vi "Logger Test Interface.vi"() -> ()   [LabVIEW 2012, in "Logger VIs.lvlib"]
uses:
  Logger VIs.lvlib
  State.ctl
panel:
  in  "Holding Potential":dbl(knob) scale=0.0..10.0
  in  "Current":dbl(knob) scale=0.0..10.0
  in  "Threshold":dbl(knob) scale=0.0..10.0
  in  "Resistance":dbl(knob) scale=0.0..10.0
  in  "Pressure":dbl(knob) scale=0.0..10.0
  out "Threshold":dbl(graph)
  out "Position":cluster{"X":dbl, "Y":dbl, "Z":dbl} {"Z" format="%.2f"; "Y" format="%.2f"; "X" format="%.2f"}
  out "Current State":T1=enum."LOAD"
  out "Holding Potential":dbl(graph)
  out "Pressure":dbl(graph)
  out "Current":dbl(graph)
  out "Resistance":dbl(graph)
  out "Full Path":path
  in  "base path":path
  out "error out":errorcluster
  in  "error in (no error)":errorcluster
  in  "Stop":bool caption="Start 2"
  out "Recording indicator":bool
  in  "Record":bool caption="Start 2"
  # "um"
  # "um"
  # "um"
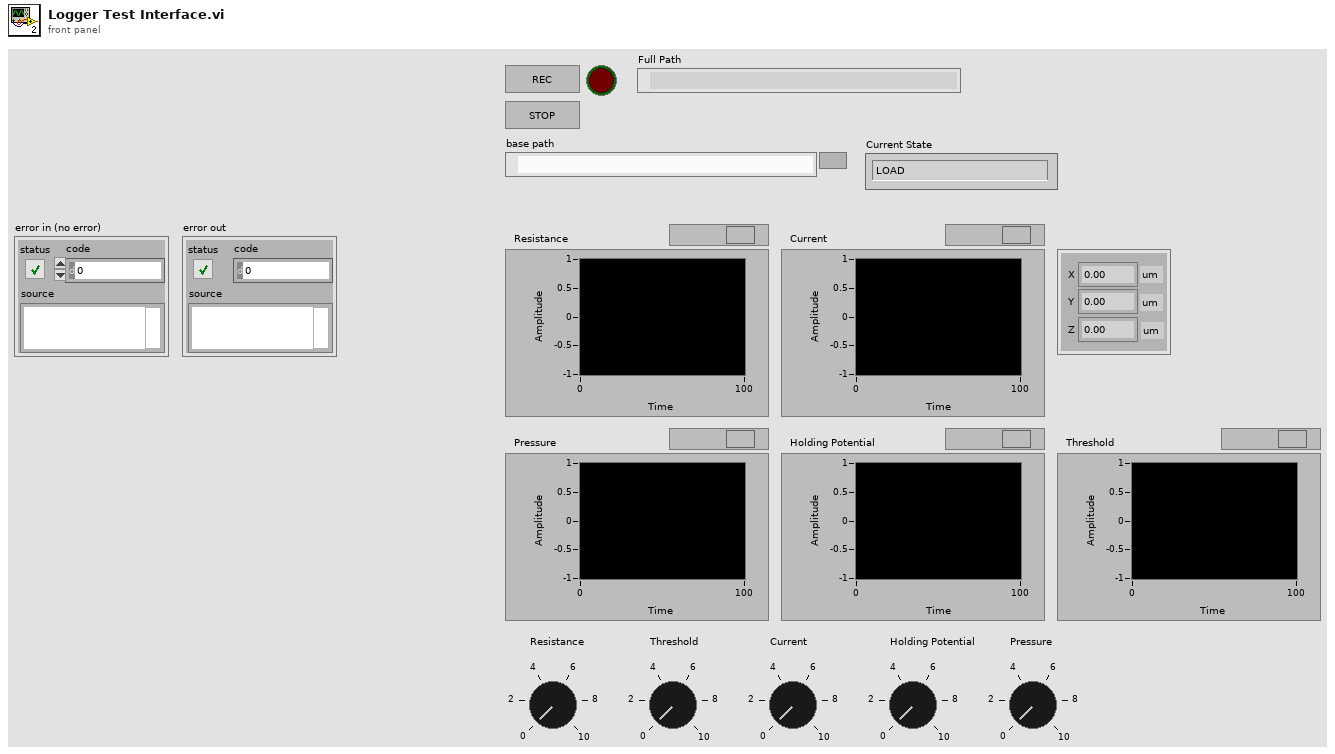
[diagram p1: front panel]
types:
  T1 = typedef "State.ctl" = enum16{"READY", "LOAD", "LOCALIZATION", "HUNTING", "SEAL", "BREAKIN", "WCR"}
  T2 = cluster{"Resistance":refnum<vi>, "Current":refnum<vi>, "Holding Potential":refnum<vi>, "Current State":refnum<vi>, "Recording indicator":refnum<vi>, "Threshold":refnum<vi>, "Pressure":refnum<vi>, "Path":refnum<vi>, "Manipulator Position":refnum<vi>}
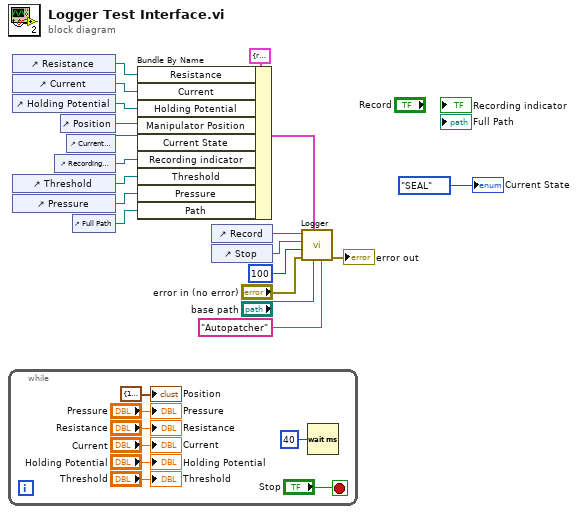
[diagram p0: block diagram]
diagram:
  n1 = while {
    stop <- "Stop" stop-if-true
    n2 = Wait (ms)(milliseconds to wait=u32 40) -> ()  [unwired: 1 out]
    "Resistance" <- "Resistance"
    "Current" <- "Current"
    "Pressure" <- "Pressure"
    "Holding Potential" <- "Holding Potential"
    "Position" <- cluster{"X":dbl, "Y":dbl, "Z":dbl} {"X"=10.0, "Y"=20.0, "Z"=30.0} ("Position")
    "Threshold" <- "Threshold"
  }
  n3 = control-ref of="Resistance"() -> (w10:refnum<vi>)
  n4 = control-ref of="Current"() -> (w9:refnum<vi>)
  n5 = control-ref of="Holding Potential"() -> (w3:refnum<vi>)
  n6 = control-ref of="Threshold"() -> (w4:refnum<vi>)
  n7 = control-ref of="Pressure"() -> (w7:refnum<vi>)
  n8 = control-ref of="Recording indicator"() -> (w8:refnum<vi>)
  n9 = control-ref of="Position"() -> (w2:refnum<vi>)
  n10 = control-ref of="Current State"() -> (w11:refnum<vi>)
  n11 = control-ref of="Full Path"() -> (w14:refnum<vi>)
  n12 = Bundle By Name(cluster=T2 {"Resistance"=refnum, "Current"=refnum, "Holding Potential"=refnum, "Current State"=refnum, "Recording indicator"=refnum, "Threshold"=refnum, "Pressure"=refnum, "Path"=refnum, "Manipulator Position"=refnum} ("Indicators"), "Resistance"=w10, "Current"=w9, "Holding Potential"=w3, "Manipulator Position"=w2, "Current State"=w11, "Recording indicator"=w8, "Threshold"=w4, "Pressure"=w7, "Path"=w14) -> (w6:T2)
  n13 = control-ref of="Record"() -> (w19:refnum<vi>)
  n14 = control-ref of="Stop"() -> (w1:refnum<vi>)
  n15 = call "Logger.vi"("Filename"="Autopatcher", "File Path Control"="base path", "Indicators"=w6, "error in (no error)"="error in (no error)", "Period [ms]"=i64 100, "Exit"=w1, "Record"=w19) -> ("error out"=→"error out":errorcluster)  [unwired: 4 in]
  "Current State" <- State."SEAL" ("Current State")
